vi "MainZSCAN.vi"() -> ()   [LabVIEW 2018]
uses:
  MainStateControls.ctl
  <vilib>/Instr/_visa.llb/VISA Configure Serial Port (Instr).vi
panel:
  out "error out":errorcluster
  out "Position (mm)":dbl
  out "number":dbl
  out "read buffer":string
  in  "HOME Button":bool
  in  "UNITS (mm)":i32 min=0 max=825
  in  "VISA resource name":refnum<visa-resource-name>
  in  "Stop Movement":bool
  in  "ZSCAN Button":bool
  in  "RIGHT Button":bool
  in  "LEFT Button":bool
  in  "stopProgrammButton":bool
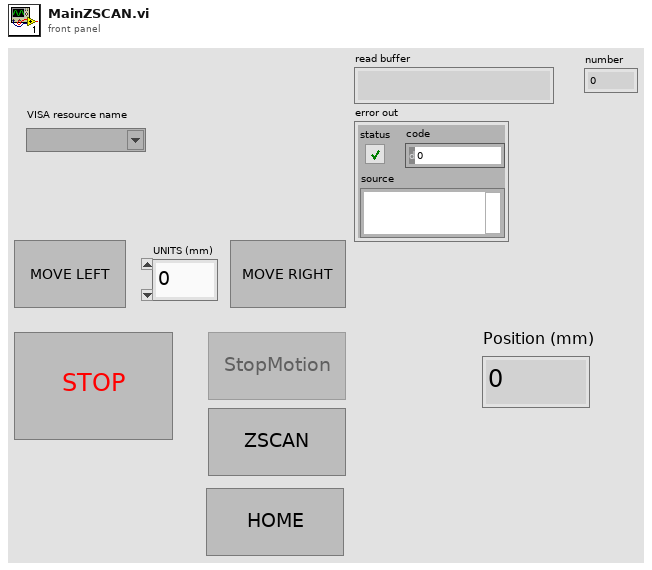
[diagram p1: front panel]
types:
  T1 = typedef "MainStateControls.ctl" = enum16{"init", "wait for event", "MoveLeft", "MoveRight", "StopMovement", "Zscan", "Home", "Read", "Stop"}
  T2 = enum8{"Enabled", "Disabled", "Disabled and Grayed Out"}
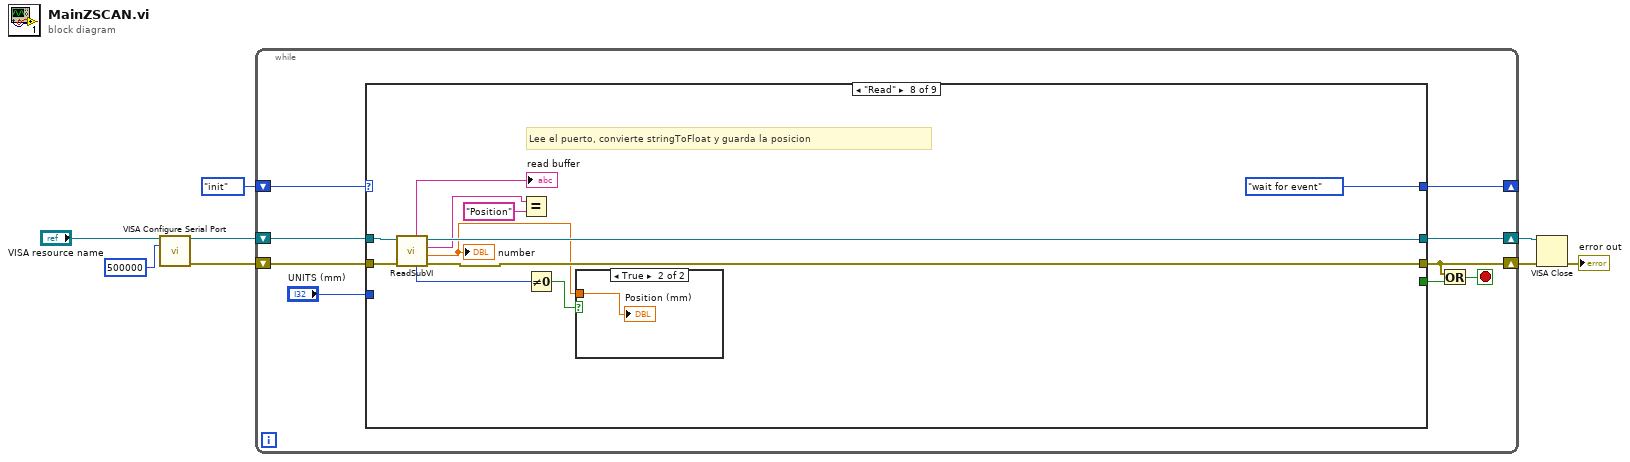
[diagram p0: block diagram]
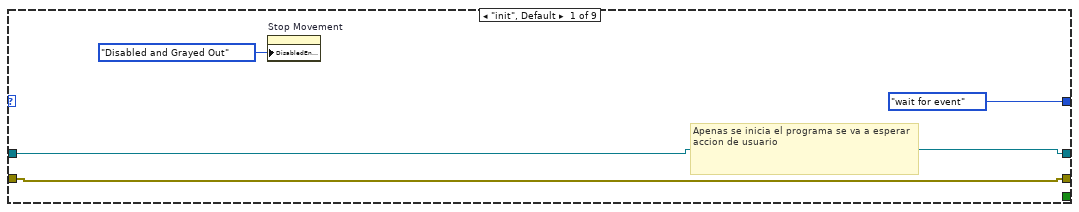
[diagram p2: hidden frame]
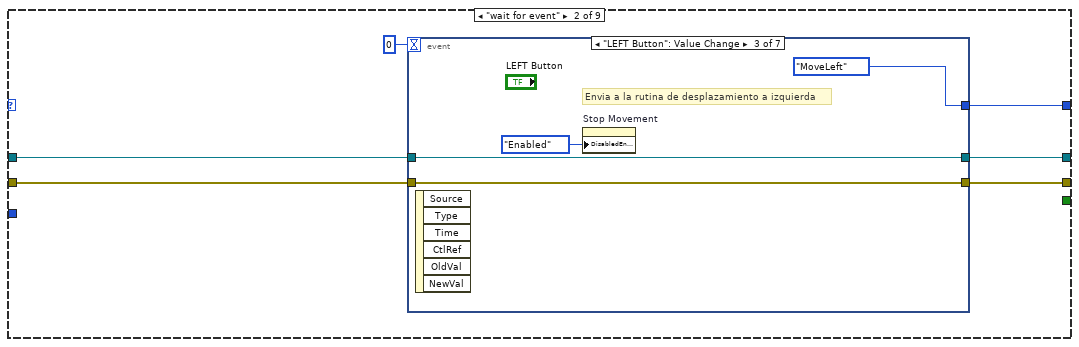
[diagram p3: hidden frame]
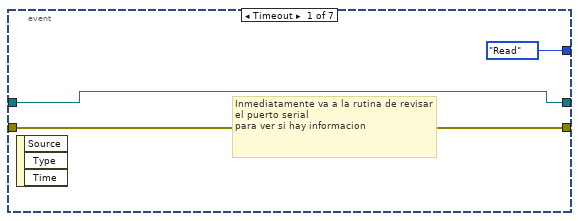
[diagram p4: hidden frame]
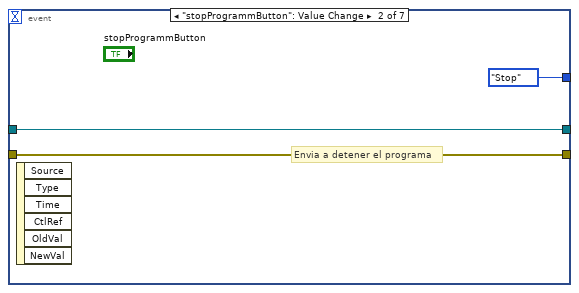
[diagram p5: hidden frame]
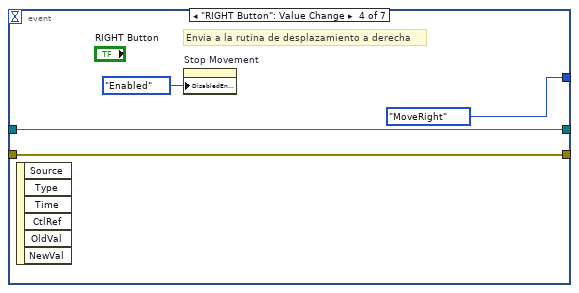
[diagram p6: hidden frame]
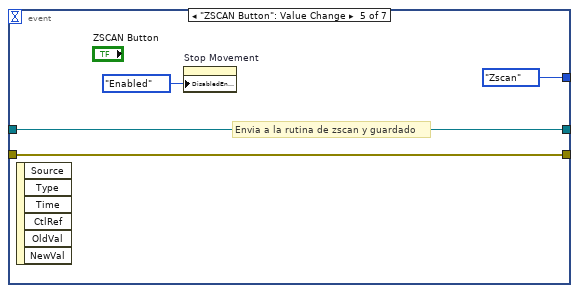
[diagram p7: hidden frame]
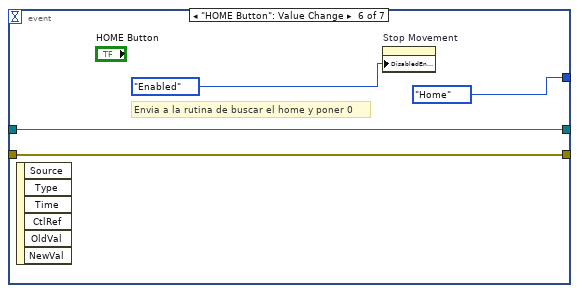
[diagram p8: hidden frame]
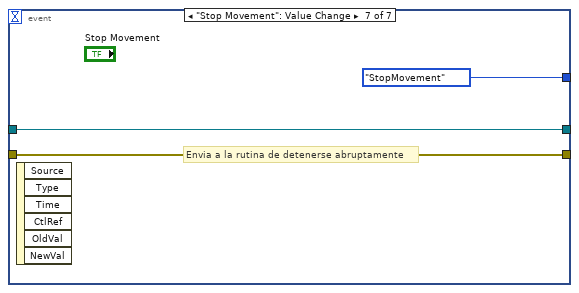
[diagram p9: hidden frame]
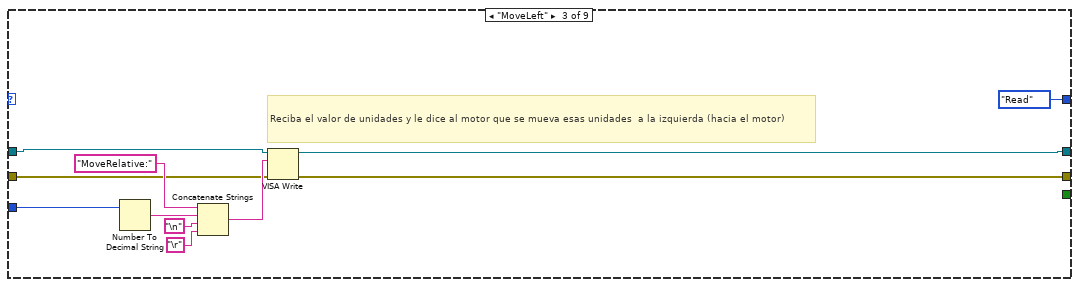
[diagram p10: hidden frame]
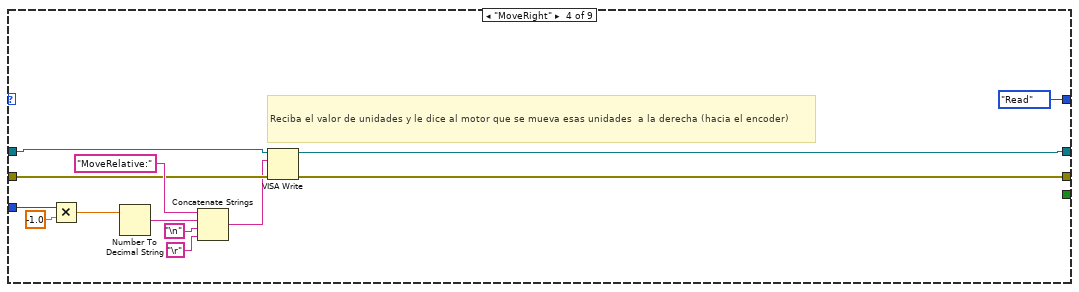
[diagram p11: hidden frame]
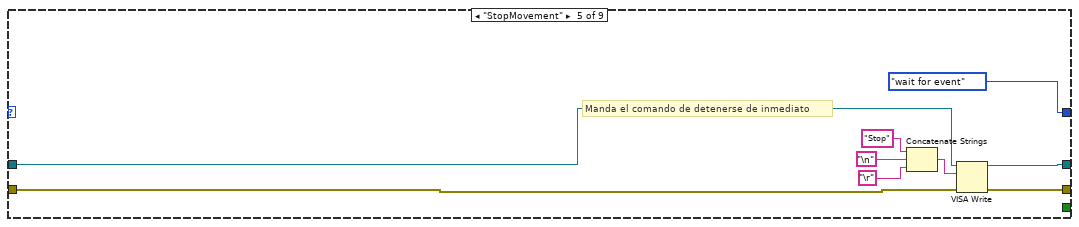
[diagram p12: hidden frame]
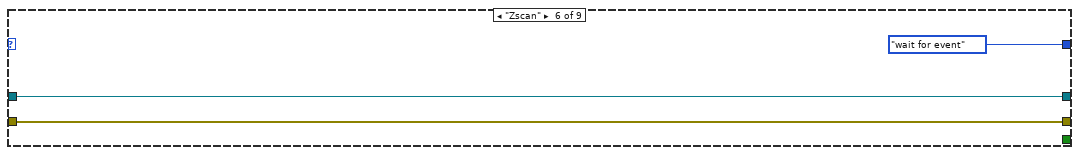
[diagram p13: hidden frame]
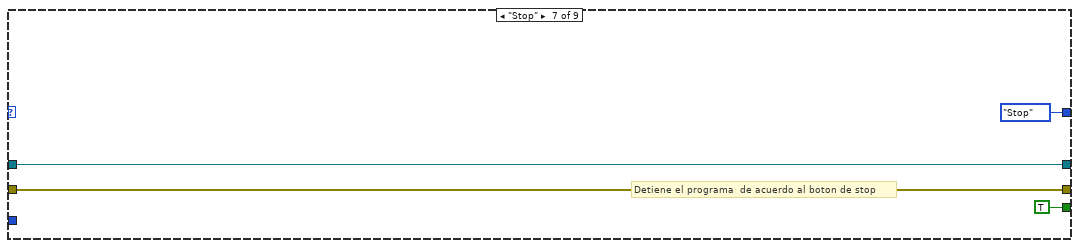
[diagram p14: hidden frame]
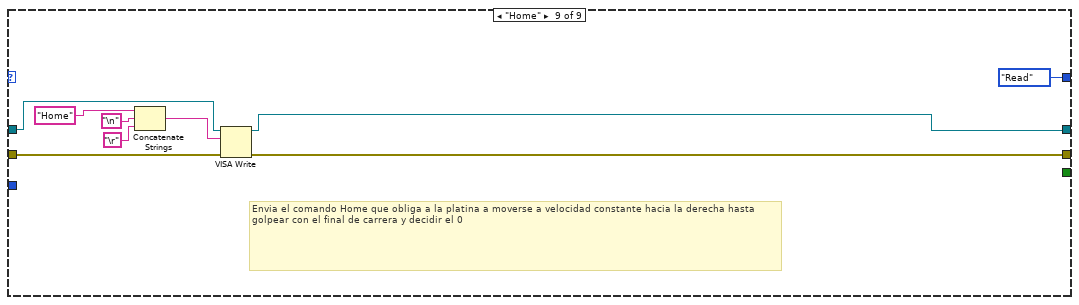
[diagram p16: hidden frame]
diagram:
  n1 = call-poly "VISA Configure Serial Port"("VISA resource name"="VISA resource name", "baud rate (9600)"=u32 500000) -> ("VISA resource name out"=w5:refnum<visa-resource-name>, "error out"=w3:errorcluster)  [unwired: 12 in]
  n2 = while {
    shift-right: [w16] -> _
    shift-left: MainStateControls."init" -> [w17]
    shift-right: [w10] -> w2
    shift-left: w3 -> [w13]
    shift-right: [w14] -> w4
    shift-left: w5 -> [w15]
    stop <- w9 stop-if-true
    n3 = case shown="\"Read\"" w17 {
      tunnel: [MainStateControls."wait for event" w26 MainStateControls."Read" MainStateControls."Read" MainStateControls."wait for event" MainStateControls."wait for event" MainStateControls."Stop" MainStateControls."wait for event" MainStateControls."Read"] -> w16
      tunnel: [_ _ _ _ _ _ TRUE _ _] -> w11
      tunnel: w15 -> [w20 w25 w59 w70 w83 w87 w90 w102 w113]
      tunnel: [w20 w24 w57 w68 w81 w87 w90 w100 w111] -> w14
      tunnel: w13 -> [w19 w23 w58 w71 w84 w86 w89 w101 w112]
      tunnel: [w19 w22 w56 w69 w82 w86 w89 w99 w110] -> w10
      tunnel: "UNITS (mm)" -> [_ _ w55 w67 _ _ _ _ _]
      frame "init", Default {
        # "Apenas se inicia el programa se va a esperar accion de usuario"
        n4 = property on="Stop Movement" class="Bool"("DisabledEnum"=T2."Disabled and Grayed Out" ("Disabled")) -> ()  [unwired: 2 in, 2 out]
      }
      frame "wait for event" {
        n5 = event shown="[2] \"LEFT Button\": Value Change" {
          selector: _ -> [_ _ _ _ _ _ _]
          dyn-events: _ -> [_ _ _ _ _ _ _]
          timeout: 0 -> [_ _ _ _ _ _ _]
          tunnel: [MainStateControls."Read" MainStateControls."Stop" MainStateControls."MoveLeft" MainStateControls."MoveRight" MainStateControls."Zscan" MainStateControls."Home" MainStateControls."StopMovement"] -> w26
          tunnel: w25 -> [w29 w32 w36 w40 w44 w48 w51]
          tunnel: [w29 w32 w36 w40 w44 w48 w51] -> w24
          tunnel: w23 -> [w28 w31 w35 w39 w43 w47 w50]
          tunnel: [w28 w31 w35 w39 w43 w47 w50] -> w22
          event Timeout {
            # "Inmediatamente va a la rutina de revisar el puerto serial\npara ver si hay informacion"
            n6 = event-data() -> ()  [unwired: 1 in, 3 out]
          }
          event "stopProgrammButton": Value Change {
            # "Envia a detener el programa"
            n7 = event-data() -> ()  [unwired: 1 in, 6 out]
          }
          event "LEFT Button": Value Change {
            # "Envia a la rutina de desplazamiento a izquierda"
            n8 = event-data() -> ()  [unwired: 1 in, 6 out]
            n9 = property on="Stop Movement" class="Bool"("DisabledEnum"=T2."Enabled" ("Disabled")) -> ()  [unwired: 2 in, 2 out]
          }
          event "RIGHT Button": Value Change {
            # "Envia a la rutina de desplazamiento a derecha"
            n10 = event-data() -> ()  [unwired: 1 in, 6 out]
            n11 = property on="Stop Movement" class="Bool"("DisabledEnum"=T2."Enabled" ("Disabled")) -> ()  [unwired: 2 in, 2 out]
          }
          event "ZSCAN Button": Value Change {
            # "Envia a la rutina de zscan y guardado"
            n12 = event-data() -> ()  [unwired: 1 in, 6 out]
            n13 = property on="Stop Movement" class="Bool"("DisabledEnum"=T2."Enabled" ("Disabled")) -> ()  [unwired: 2 in, 2 out]
          }
          event "HOME Button": Value Change {
            # "Envia a la rutina de buscar el home y poner 0"
            n14 = event-data() -> ()  [unwired: 1 in, 6 out]
            n15 = property on="Stop Movement" class="Bool"("DisabledEnum"=T2."Enabled" ("Disabled")) -> ()  [unwired: 2 in, 2 out]
          }
          event "Stop Movement": Value Change {
            # "Envia a la rutina de detenerse abruptamente"
            n16 = event-data() -> ()  [unwired: 1 in, 6 out]
          }
        }
      }
      frame "MoveLeft" {
        # "Reciba el valor de unidades y le dice al motor que se mueva esas unidades  a la izquierda (hacia el motor)"
        n17 = Number To Decimal String(number=w55) -> (decimal integer string=w61:string)  [unwired: 1 in]
        n18 = Concatenate Strings("MoveRelative:", w61, "\n", "\r") -> (w62:string)
        n19 = VISA Write(VISA resource name=w59, write buffer=w62, error in (no error)=w58) -> (VISA resource name out=w57:refnum<visa-resource-name>, error out=w56:errorcluster)  [unwired: 1 out]
      }
      frame "MoveRight" {
        # "Reciba el valor de unidades y le dice al motor que se mueva esas unidades  a la derecha (hacia el encoder)"
        n20 = Multiply(x=w67, y=-1.0) -> (x*y=w72:dbl)
        n21 = Number To Decimal String(number=w72) -> (decimal integer string=w74:string)  [unwired: 1 in]
        n22 = Concatenate Strings("MoveRelative:", w74, "\n", "\r") -> (w66:string)
        n23 = VISA Write(VISA resource name=w70, write buffer=w66, error in (no error)=w71) -> (VISA resource name out=w68:refnum<visa-resource-name>, error out=w69:errorcluster)  [unwired: 1 out]
      }
      frame "StopMovement" {
        # "Manda el comando de detenerse de inmediato"
        n24 = Concatenate Strings("Stop" ("write buffer"), "\n", "\r") -> (w77:string)
        n25 = VISA Write(VISA resource name=w83, write buffer=w77, error in (no error)=w84) -> (VISA resource name out=w81:refnum<visa-resource-name>, error out=w82:errorcluster)  [unwired: 1 out]
      }
      frame "Zscan" {
      }
      frame "Stop" {
        # "Detiene el programa  de acuerdo al boton de stop"
      }
      frame "Read" {
        # "Lee el puerto, convierte stringToFloat y guarda la posicion"
        n26 = call "ReadSubVI.vi"("error in (no error)"=w101, "reference"=w102) -> ("error out"=w99:errorcluster, "number"=w94:dbl, "before substring"=w96:string, "VISA resource name out"=w100:refnum<visa-resource-name>, "Bytes at port"=w97:u32, "read buffer"=→"read buffer":string)  [unwired: 4 in]
        "number" <- w94
        n27 = Equal?(x=w96, y="Position") -> ()  [unwired: 1 out]
        n28 = Not Equal To 0?(x=w97) -> (x != 0?=w93:bool)
        n29 = case shown="True" w93 {
          tunnel: w94 -> [_ w104]
          frame False {
          }
          frame True {
            "Position (mm)" <- w104
          }
        }
      }
      frame "Home" {
        # "Envia el comando Home que obliga a la platina a moverse a velocidad constante hacia la derecha hasta golpear con el final de carrera y decidir el 0"
        n30 = Concatenate Strings("Home" ("write buffer"), "\n", "\r") -> (w105:string)
        n31 = VISA Write(VISA resource name=w113, write buffer=w105, error in (no error)=w112) -> (VISA resource name out=w111:refnum<visa-resource-name>, error out=w110:errorcluster)  [unwired: 1 out]
      }
    }
    n32 = Or(x=w10, y=w11) -> (x .or. y?=w9:bool)
  }
  n33 = VISA Close(VISA resource name=w4, error in (no error)=w2) -> (error out=→"error out":errorcluster)
